vi "Dashboard.vi"() -> (3 "Overlay state":bool)   [LabVIEW 2016]
uses:
  Globals/InputValues.vi
  Globals/Globals.vi
  Globals/Constantes.vi
  <vilib>/Rock Robotics/Network Tables/NT Write Number.vi
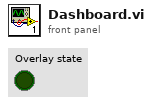
[diagram p1: front panel]
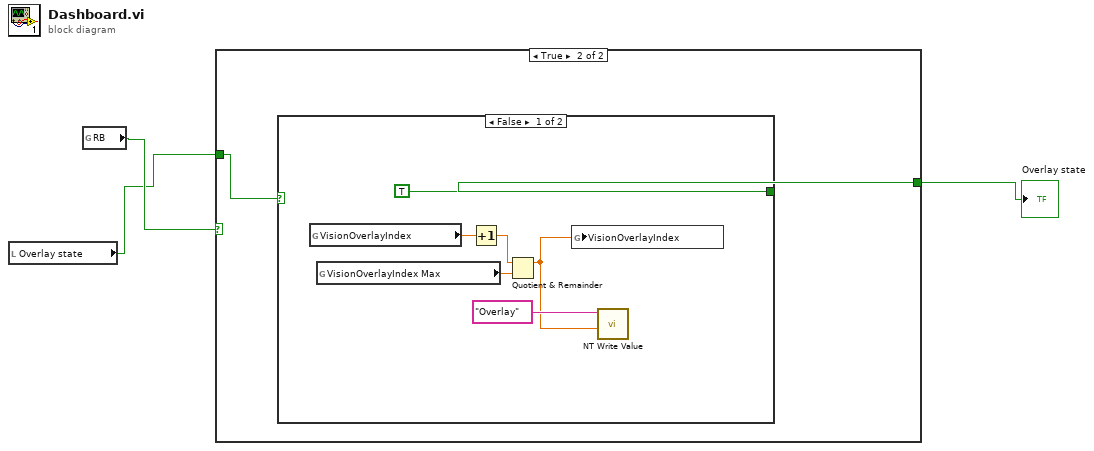
[diagram p0: block diagram]
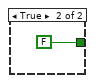
[diagram p3: hidden frame]
diagram:
  n1 = local read "Overlay state"() -> (w1:bool)
  n2 = global read "InputValues.vi" "RB"() -> (w2:bool)
  n3 = case shown="True" w2 {
    tunnel: w1 -> [w5 w9]
    tunnel: [w4 w8] -> w3
    frame False {
      n4 = case shown="False" w5 {
        selector: w5 -> [w6 _]
        tunnel: [w6 FALSE] -> w4
        frame False {
        }
        frame True {
        }
      }
    }
    frame True {
      n5 = case shown="False" w9 {
        selector: w9 -> [_ w16]
        tunnel: [TRUE w16] -> w8
        frame False {
          n6 = global read "Globals.vi" "VisionOverlayIndex"() -> (w14:dbl)
          n7 = global read "Constantes.vi" "VisionOverlayIndex Max"() -> (w13:dbl)
          n8 = Increment(x=w14) -> (x+1=w11:dbl)
          n9 = Quotient & Remainder(x=w11, y=w13) -> (x-y*floor(x/y)=w10:dbl)  [unwired: 1 out]
          n10 = global write "Globals.vi" "VisionOverlayIndex"(w10) -> ()
          n11 = call-poly <vilib>:"NT Write Value.vi"("Numeric"=w10, "Name"="Overlay") -> ()  [unwired: 9 in, 1 out]
        }
        frame True {
        }
      }
    }
  }
  "Overlay state" <- w3
